vi "OAT Torsional Vibration (Digital Tacho) (Even-Angle) (N Ch - 1 Setting).vi"(0 "digital tacho info":T7[](array[typedef]), 2 "pulse/revolution (1)":i32=1 min=1, 4 "torsional vibration units":enum16{"RPM", "deg/s", "rad/s"}(ring), 5 "error in (no error)":errorcluster, 8 "reset? (F)":bool) -> (14 "even-angle torsional vibration signals":cluster{"r0":dbl, "dr":dbl, "Y":dbl[]}[](array[cluster]) {"r0" format="%.2p"; "dr" format="%.2p"; "Y" format="%.2f"}, 15 "even-angle channel info":T3[](array[typedef]) {"channel info"."pregain" format="%.2f"; "channel info"."weighting filter" items=["Linear", "A-weighting", "B-weighting", "C-weighting", "ITU-R 468-4", "Dolby", "CCITT", "C-message", "Wb", "Wc", "Wd", "We", "Wf", "Wh", "Wj", "Wk", "Wm", "AES17 20 kHz lowpass", "AES17 40 kHz lowpass", "AES17 20 kHz highpass", "AES17 40 kHz highpass"]; "channel info"."dB reference" format="%^.1e"; "channel info"."engineering units" items=["custom..."=0, "V"=1, "A"=21, "C"=30, "pC"=31, "s"=32, "-"=29, "Pa"=2, "N"=20, "g"=3, "m/s^2"=4, "m/s"=5, "m"=6, "mm/s"=12, "mm"=13, "micron/s"=14, "micron"=15, "in/s^2"=7, "in/s"=8, "in"=9, "mil/s"=10, "mil"=11, "rad/s^2"=16, "rad/s"=17, "rad"=18, "deg/s^2"=26, "deg/s"=27, "deg"=28, "RPM"=22, "cycle/s^2"=23, "Hz"=24, "cycle"=25, "strain"=19]; "channel info"."sensor sensitivity" format="%#_5f"}, 16 "speed profiles":T2[](array[typedef]) {"speed [RPM]" format="%.2f"; "time [s]" format="%.2f"}, 17 "position info":T1[](array[typedef]), 18 "unit labels":string[](array[string]), 19 "error out":errorcluster)   [LabVIEW 2017, in "SoundVib_Torsional.lvlib"]
doc: "Calculates torsional vibration signals from digital tachometer signals. This VI can return torsional vibration signals as either waveform signals or even-angle signals. Wire data to the <B>digital tacho info</B> input to determine the polymorphic instance to use or manually select the instance."
uses:
  <vilib>/addons/Sound and Vibration/Order Analysis/Torsional Vibration/SoundVib_Torsional.lvlib
  <vilib>/addons/Sound and Vibration/Order Analysis/Tach Process/SubVIs/digital tach info.ctl
  <vilib>/addons/_NISVFA/_Shared subVIs/Controls/svc_Resampled Channel Info.ctl
  <vilib>/addons/_NISVFA/_Shared subVIs/Controls/svc_Channel Info.ctl
  <vilib>/addons/_NISVFA/_Shared subVIs/Controls/svc_Engineering Units Text Ring.ctl
  <vilib>/addons/_NISVFA/_Shared subVIs/Controls/svc_Weighting Filter Text Ring.ctl
  <vilib>/addons/Sound and Vibration/Order Analysis/Tach Process/SubVIs/speed profile.ctl
  <vilib>/addons/Sound and Vibration/Order Analysis/Misc/OAT Position Info.ctl
  <vilib>/addons/Sound and Vibration/Order Analysis/Tach Process/SoundVib_TachProcess.lvlib
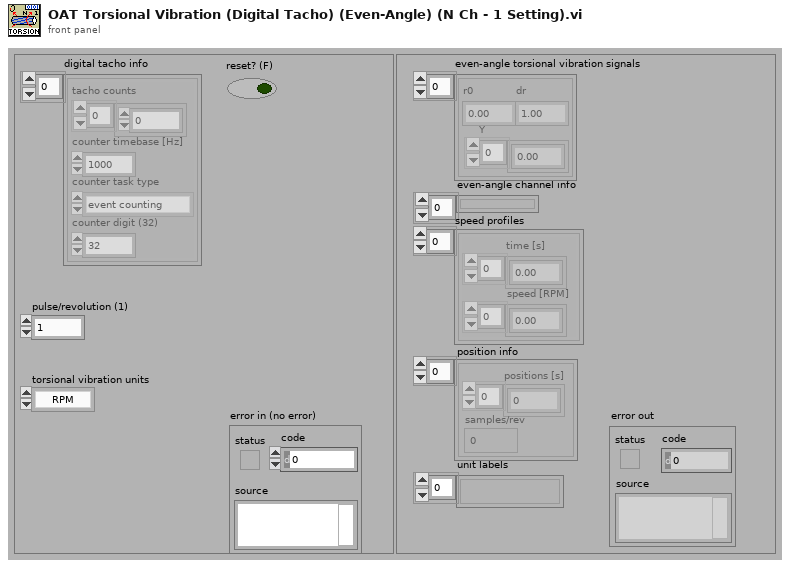
[diagram p1: front panel]
types:
  T1 = typedef "OAT Position Info.ctl" = cluster{"positions [s]":dbl[], "samples/rev":dbl}
  T2 = typedef "SoundVib_TachProcess.lvlib/speed profile.ctl" = cluster{"time [s]":dbl[], "speed [RPM]":dbl[]}
  T3 = typedef "svc_Resampled Channel Info.ctl" = cluster{"channel name":string, "description":string, " channel info":T4}
  T4 = typedef "svc_Channel Info.ctl" = cluster{"sensor sensitivity":dbl, "engineering units":T5, "dB reference":dbl, "custom label":string, "weighting filter":T6, "pregain":dbl}
  T5 = typedef "svc_Engineering Units Text Ring.ctl" = u16
  T6 = typedef "svc_Weighting Filter Text Ring.ctl" = u16
  T7 = typedef "SoundVib_TachProcess.lvlib/digital tach info.ctl" = cluster{"tacho counts":i64[], "counter timebase [Hz]":dbl, "counter task type":enum16{"period measurement", "event counting"}, "counter digit (32)":i32}
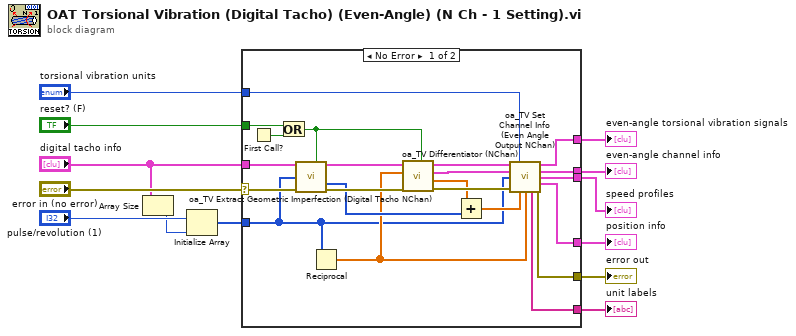
[diagram p0: block diagram]
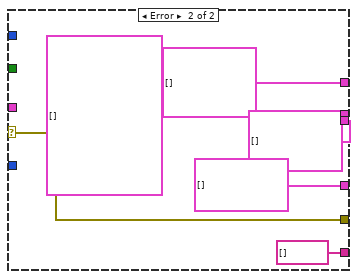
[diagram p2: hidden frame]
diagram:
  n1 = Array Size(array="digital tacho info") -> (size(s)=w4:i32)
  n2 = Initialize Array("pulse/revolution (1)", w4) -> (w3:i32[])
  n3 = case shown="No Error" "error in (no error)" {
    selector: "error in (no error)" -> [w28 w41]
    tunnel: "reset? (F)" -> [w32 _]
    tunnel: "digital tacho info" -> [w29 _]
    tunnel: w3 -> [w17 _]
    tunnel: "torsional vibration units" -> [w20 _]
    tunnel: [w23 T3[] [] ("even-angle channel info")] -> w10
    tunnel: [w22 cluster{"r0":dbl, "dr":dbl, "Y":dbl[]}[] [] ("even-angle torsional vibration")] -> w9
    tunnel: [w26 w41] -> w11
    tunnel: [w19 string[] [] ("unit labels")] -> w7
    tunnel: [w16 T2[] [] ("speed profiles")] -> w2
    tunnel: [w15 T1[] [] ("position info")] -> w1
    frame No Error {
      n4 = First Call?() -> (First Call?: T/F=w33:bool)
      n5 = Or(x=w32, y=w33) -> (x .or. y?=w30:bool)
      n6 = call <vilib>:"oa_TV Extract Geometric Imperfection (Digital Tacho NChan).vi"("digital tacho info"=w29, "reset? (F)"=w30, "pulse/revolution"=w17, "error in (no error)"=w28) -> ("pulse positions"=w31:cluster{dbl[]}[], "revulotion index"=w34:i32[], "error out"=w35:errorcluster)  [unwired: 8 in, 1 out]
      n7 = Reciprocal(x=w17) -> (1/x=w25:dbl[])
      n8 = call <vilib>:"oa_TV Differentiator (NChan).vi"("reset? (False)"=w30, "error in (no error)"=w35, "delta X"=w25, "Y[n]"=w31) -> ("error out"=w27:errorcluster, "Delay"=w14:dbl[], "X[n]"=w18:cluster{dbl[]}[], "dY[n]/dX[n]"=w21:cluster{dbl[]}[])  [unwired: 4 in]
      n9 = Add(x=w14, y=w34) -> (x+y=w24:dbl[])
      n10 = call <vilib>:"oa_TV Set Channel Info (Even Angle Output NChan).vi"("seconds/revolution"=w21, "torisional vibration unit (RPM)"=w20, "pulse positions"=w18, "pulse/revolution (1)"=w17, "error in (no error)"=w27, "r0"=w24, "dr"=w25) -> ("even-angle torsional vibration"=w22:cluster{"r0":dbl, "dr":dbl, "Y":dbl[]}[], "even-angle channel info"=w23:T3[], "speed profiles"=w16:T2[], "position info"=w15:T1[], "unit labels"=w19:string[], "error out"=w26:errorcluster)  [unwired: 3 in]
    }
    frame Error {
    }
  }
  "error out" <- w11
  "even-angle channel info" <- w10
  "even-angle torsional vibration signals" <- w9
  "unit labels" <- w7
  "speed profiles" <- w2
  "position info" <- w1
